vi "Optionen_BoolenControls.vi"(8 "error in (no error)":errorcluster caption="Fehler (Eingang, kein Fehler)", 11 "Controls[]":refnum<vi>[](array[refnum])) -> (0 "error out":errorcluster caption="Fehler (Ausgang)", 3 "BooleanControls[] (Ausgang)":refnum<vi>[](array[refnum]))   [LabVIEW 2020, in "System Einstellungen V2.lvlib"]
uses:
  System Einstellungen V2.lvlib
  <vilib>/Utility/Data Type/NI_Data Type.lvlib
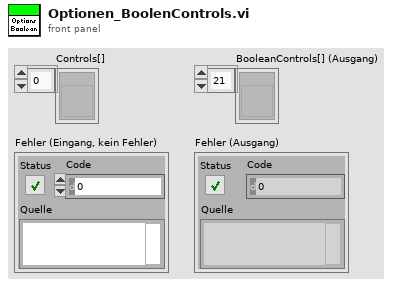
[diagram p1: front panel]
types:
  T1 = typedef "NI_Data Type.lvlib/Data Type.ctl" = enum8{"Invalid Type", "Void", "I8", "I16", "I32", "I64", "U8", "U16", "U32", "U64", "Single Float", "Double Float", "Extended Float", "Single Complex", "Double Complex", "Extended Complex", "Enum U8", "Enum U16", "Enum U32", "Enum U64", "Single Float With Unit", "Double Float With Unit", "Extended Float With Unit", "Single Complex with Unit", "Double Complex with Unit", "Extended Complex with Unit", "Boolean", "String", "Path", "Picture", "Tag", "Array", "Cluster", "Variant", "LV Variant", "Waveform", "Timestamp", "Digital Waveform", "Digital Data", "ExpressData", "Refnum", "External Data", "VI", "Poly VI", "LabVIEW Class Instance", "Fixed Point", "Set Collection", "Map Collection"}
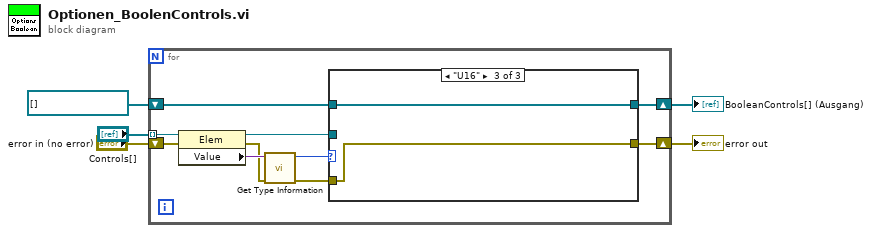
[diagram p0: block diagram]
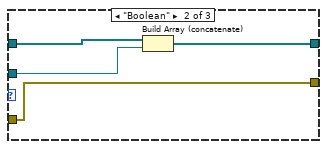
[diagram p3: hidden frame]
diagram:
  n1 = for {
    shift-right: [w9] -> w2
    shift-left: "error in (no error)" -> [w15]
    tunnel: "Controls[]" -> [w8] mode=indexing
    shift-right: [w7] -> w5
    shift-left: refnum<vi>[] [] -> [w6]
    n2 = property class="Elem"(reference=w8, error in=w15) -> (reference out=w11:refnum<vi>, error out=w12:errorcluster, "Value"=w14:variant)
    n3 = call <vilib>:"Get Type Information.vi"("error in (no error)"=w12, "variant"=w14) -> ("error out"=w10:errorcluster, "type"=w13:T1)  [unwired: 5 in, 3 out]
    n4 = case shown="\"U16\"" w13 {
      tunnel: w11 -> [_ w20 _]
      tunnel: w10 -> [w17 w18 w22]
      tunnel: [w17 w18 w22] -> w9
      tunnel: [w16 w21 w23] -> w7
      tunnel: w6 -> [w16 w19 w23]
      frame "Invalid Type", Default {
      }
      frame "Boolean" {
        n5 = Build Array (concatenate)(w19, w20) -> (w21:refnum<vi>[])
      }
      frame "U16" {
      }
    }
  }
  "BooleanControls[] (Ausgang)" <- w5
  "error out" <- w2
